vi "process raw.vi"(0 "file_in":string, 1 "store_raw":bool, 2 "format_hdf":bool, 3 "csv_delimiter":i8, 5 "calibration_file":string, 7 "nFiles":i32, 9 "file_out":string, 12 "store_si":bool, 13 "compress":bool, 14 "progress":T1) -> (4 "file_in out":string, 6 "calibration_file out":string, 8 "progress out":T1, 10 "function return":i32)   [LabVIEW 2019, in "apdm.lvlib"]
doc: "APDM_EXPORT int apdm_process_raw(char **file_in, char **calibration_file, int nFiles, const char *file_out, const bool store_raw, const bool store_si, const bool format_hdf, const bool compress, char csv_delimiter, apdm_progress_t *progress);"
uses:
  apdm.lvlib
  Lee Lab/CP FES Walking 2018/Code/Working/LabVIEW/apdm.dll
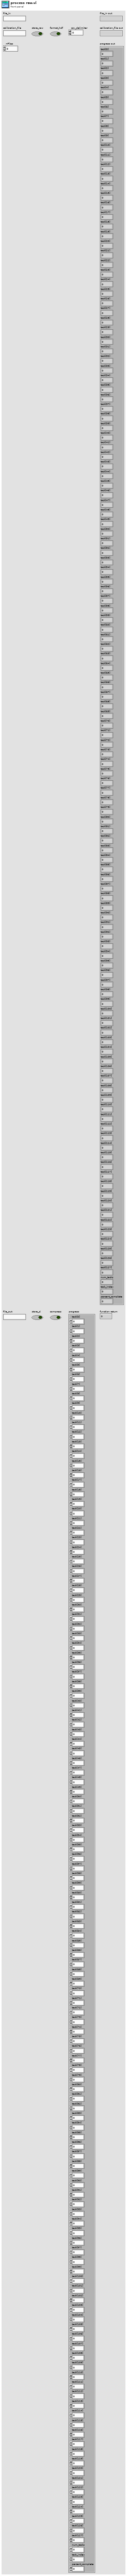
[diagram p1: front panel]
types:
  T1 = cluster{"task[0]":i8, "task[1]":i8, "task[2]":i8, "task[3]":i8, "task[4]":i8, "task[5]":i8, "task[6]":i8, "task[7]":i8, "task[8]":i8, "task[9]":i8, "task[10]":i8, "task[11]":i8, "task[12]":i8, "task[13]":i8, "task[14]":i8, "task[15]":i8, "task[16]":i8, "task[17]":i8, "task[18]":i8, "task[19]":i8, "task[20]":i8, "task[21]":i8, "task[22]":i8, "task[23]":i8, "task[24]":i8, "task[25]":i8, "task[26]":i8, "task[27]":i8, "task[28]":i8, "task[29]":i8, "task[30]":i8, "task[31]":i8, "task[32]":i8, "task[33]":i8, "task[34]":i8, "task[35]":i8, "task[36]":i8, "task[37]":i8, "task[38]":i8, "task[39]":i8, "task[40]":i8, "task[41]":i8, "task[42]":i8, "task[43]":i8, "task[44]":i8, "task[45]":i8, "task[46]":i8, "task[47]":i8, "task[48]":i8, "task[49]":i8, "task[50]":i8, "task[51]":i8, "task[52]":i8, "task[53]":i8, "task[54]":i8, "task[55]":i8, "task[56]":i8, "task[57]":i8, "task[58]":i8, "task[59]":i8, "task[60]":i8, "task[61]":i8, "task[62]":i8, "task[63]":i8, "task[64]":i8, "task[65]":i8, "task[66]":i8, "task[67]":i8, "task[68]":i8, "task[69]":i8, "task[70]":i8, "task[71]":i8, "task[72]":i8, "task[73]":i8, "task[74]":i8, "task[75]":i8, "task[76]":i8, "task[77]":i8, "task[78]":i8, "task[79]":i8, "task[80]":i8, "task[81]":i8, "task[82]":i8, "task[83]":i8, "task[84]":i8, "task[85]":i8, "task[86]":i8, "task[87]":i8, "task[88]":i8, "task[89]":i8, "task[90]":i8, "task[91]":i8, "task[92]":i8, "task[93]":i8, "task[94]":i8, "task[95]":i8, "task[96]":i8, "task[97]":i8, "task[98]":i8, "task[99]":i8, "task[100]":i8, "task[101]":i8, "task[102]":i8, "task[103]":i8, "task[104]":i8, "task[105]":i8, "task[106]":i8, "task[107]":i8, "task[108]":i8, "task[109]":i8, "task[110]":i8, "task[111]":i8, "task[112]":i8, "task[113]":i8, "task[114]":i8, "task[115]":i8, "task[116]":i8, "task[117]":i8, "task[118]":i8, "task[119]":i8, "task[120]":i8, "task[121]":i8, "task[122]":i8, "task[123]":i8, "task[124]":i8, "task[125]":i8, "task[126]":i8, "task[127]":i8, "num_tasks":i32, "task_index":i32, "percent_complete":dbl}
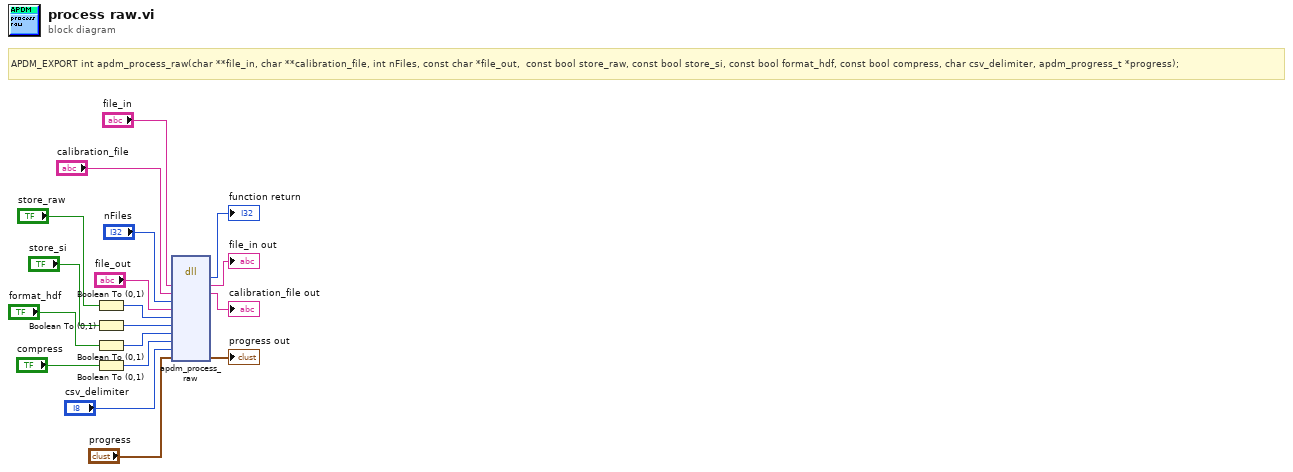
[diagram p0: block diagram]
diagram:
  # "APDM_EXPORT int apdm_process_raw(char **file_in, char **calibration_file, int nFiles, const char *file_out,  const bool store_raw, const bool store_si, const bool format_hdf, const bool compress, char csv_delimiter, apdm_progress_t *progress);"
  n1 = Boolean To (0,1)(Boolean="store_raw") -> (0, 1=w10:i16)
  n2 = Boolean To (0,1)(Boolean="store_si") -> (0, 1=w8:i16)
  n3 = Boolean To (0,1)(Boolean="format_hdf") -> (0, 1=w6:i16)
  n4 = Boolean To (0,1)(Boolean="compress") -> (0, 1=w4:i16)
  n5 = dll-call lib="C:/Users/jfalesi/Dropbox/Lee Lab/CP FES Walking 2018/Code/Working/LabVIEW/apdm.*" fn="apdm_process_raw"("file_in"="file_in", "calibration_file"="calibration_file", "nFiles"="nFiles", "file_out"="file_out", "store_raw"=w10, "store_si"=w8, "format_hdf"=w6, "compress"=w4, "csv_delimiter"="csv_delimiter", "progress"="progress") -> (→"function return":i32, "file_in"=→"file_in out":string, "calibration_file"=→"calibration_file out":string, "progress"=→"progress out":T1)  [unwired: 10 in, 2 out]
